vi "Query.vi"(6 "ISOBUS address":T1=-1 caption="ISOBUS address (-1)", 8 "error in":errorcluster, 9 "byte count":u32=4096 caption="byte count (4096)", 10 "Command":string, 11 "Mercury Reference In":T2) -> (0 "error out":errorcluster, 1 "Valid?":bool, 2 "Data":string, 3 "Mercury Reference Out":T2)   [LabVIEW 2019, in "Mercury iXX.lvlib"]
uses:
  Mercury iXX.lvlib
  Public/Controls/Mercury Reference.ctl
  Public/Controls/Comms Transport Layer.ctl
  Controls/Query Dynamic Reference.ctl
  Public/Controls/ISOBus Address.ctl
  <vilib>/Utility/error.llb/whitespace.ctl
  <vilib>/regexp/Match Regular Expression.xnode
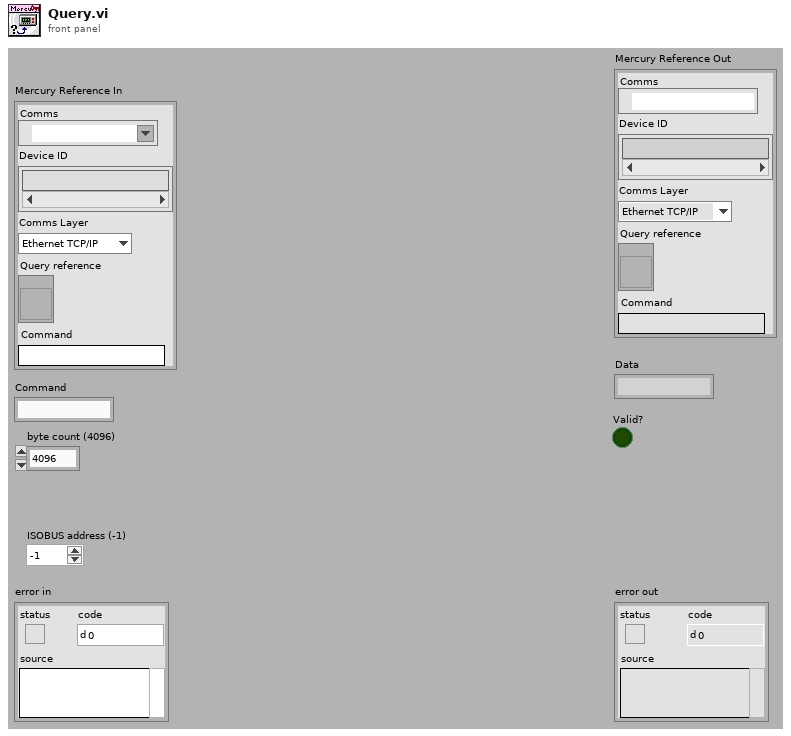
[diagram p1: front panel]
types:
  T1 = typedef "Mercury iXX.lvlib/ISOBus Address.ctl" = i32
  T2 = typedef "Mercury iXX.lvlib/Mercury Reference.ctl" = cluster{"Comms":refnum<visa-resource-name>, "Device ID":string[], "Comms Layer":T3, "Command":string, "Query reference":T4}
  T3 = typedef "Mercury iXX.lvlib/Comms Transport Layer.ctl" = enum16{"Ethernet TCP/IP", "USB", "ISOBus - RS-232", "GPIB"}
  T4 = typedef "Mercury iXX.lvlib/Query Dynamic Reference.ctl" = refnum<vi>
  T5 = typedef "whitespace.ctl" = u16
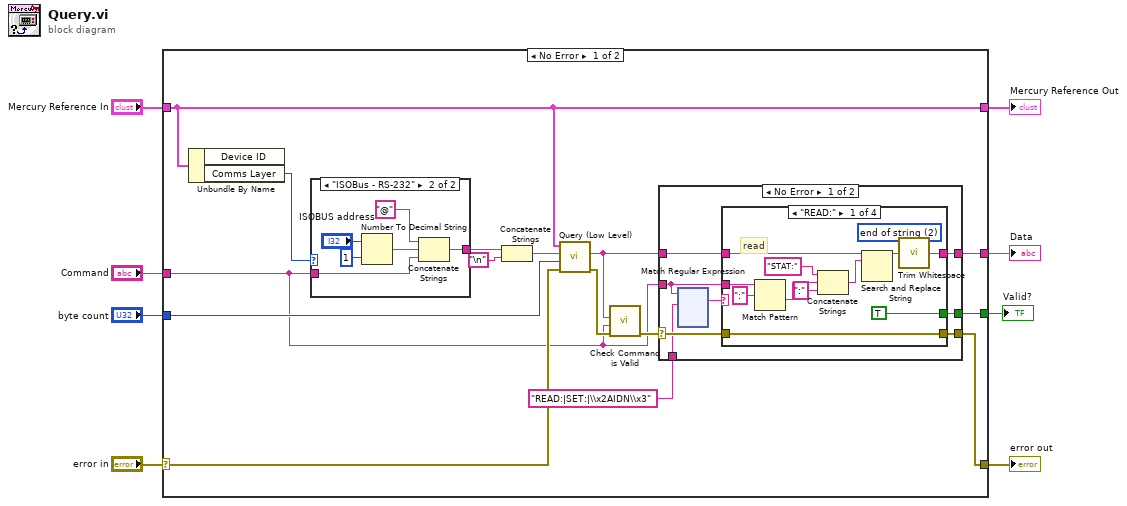
[diagram p0: block diagram]
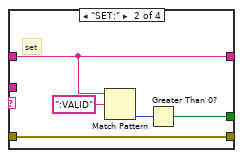
[diagram p2: hidden frame]
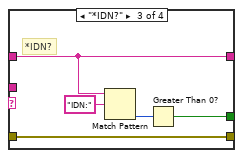
[diagram p3: hidden frame]
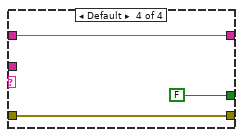
[diagram p4: hidden frame]
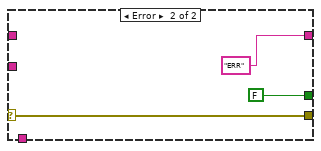
[diagram p5: hidden frame]
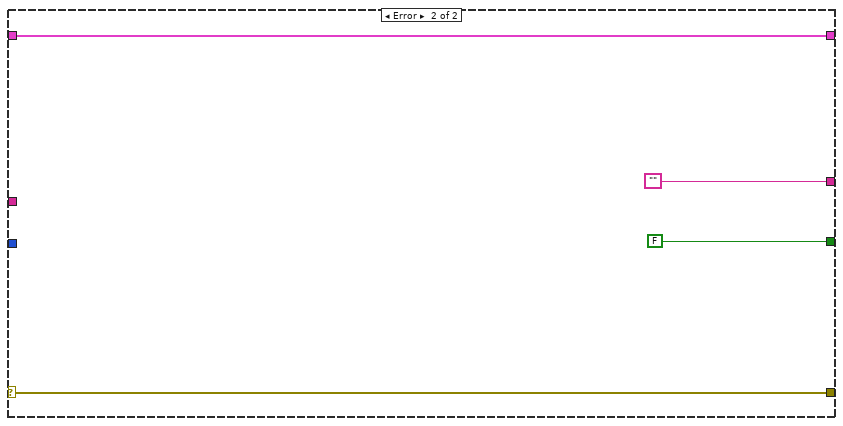
[diagram p7: hidden frame]
diagram:
  n1 = case shown="No Error" "error in" {
    selector: "error in" -> [w20 w184]
    tunnel: [w15 w184] -> w7
    tunnel: "Mercury Reference In" -> [w10 w183]
    tunnel: [w10 w183] -> w5
    tunnel: "Command" -> [w9 _]
    tunnel: [w19 ""] -> w3
    tunnel: "byte count" -> [w14 _]
    tunnel: [w13 FALSE] -> w1
    frame No Error {
      n2 = Unbundle By Name(w10) -> ("Comms Layer"=w11:T3)  [unwired: 1 out]
      n3 = case shown="\"ISOBus - RS-232\"" w11 {
        tunnel: w9 -> [w174 w176]
        tunnel: [w174 w175] -> w22
        frame "Ethernet TCP/IP", Default {
        }
        frame "ISOBus - RS-232" {
          n4 = Number To Decimal String(number="ISOBUS address", width (-)=i16 1) -> (decimal integer string=w178:string)
          n5 = Concatenate Strings("@" ("string"), w178, w176) -> (w175:string)
        }
      }
      n6 = Concatenate Strings(w22, "\n") -> (w21:string)
      n7 = call "Query (Low Level).vi"("error in"=w20, "byte count"=w14, "Command"=w21, "Mercury Reference In"=w10) -> ("error out"=w17:errorcluster, "Response"=w18:string)  [unwired: 1 in, 5 out]
      n8 = call "Check Command is Valid.vi"("error in"=w17, "Cmd Sent"=w9, "Cmd Response"=w18) -> ("error out"=w16:errorcluster)  [unwired: 8 out]
      n9 = case shown="No Error" w16 {
        selector: w16 -> [w30 w172]
        tunnel: w9 -> [w26 _]
        tunnel: [w31 "ERR" ("read buffer")] -> w19
        tunnel: w18 -> [w27 _]
        tunnel: [w29 w172] -> w15
        tunnel: [w28 FALSE] -> w13
        tunnel: "READ:|SET:|\\x2AIDN\\x3" ("regular expression") -> [w25 _]
        frame No Error {
          n10 = xnode "Match Regular Expression"("input string"=w26, "regular expression"=w25) -> ("whole match"=w24:string)  [unwired: 2 in, 6 out]
          n11 = case shown="\"READ:\"" w24 {
            tunnel: [w147 w158 w163 w168] -> w31
            tunnel: w30 -> [w154 w161 w166 w170]
            tunnel: [w154 w161 w166 w170] -> w29
            tunnel: [TRUE w160 w165 FALSE] -> w28
            tunnel: w27 -> [w151 w158 w163 w168]
            tunnel: w26 -> [w152 _ _ _]
            frame "READ:" {
              w146 = T5 2 items=["both", "start of string", "end of string"] ("location (both)")
              # "read"
              n12 = Match Pattern(string=w152, regular expression=":") -> (after substring=w156:string)  [unwired: 4 out]
              n13 = Concatenate Strings("STAT:" ("string"), w156, ":" ("string")) -> (w149:string)
              n14 = Search and Replace String(input string=w151, search string=w149) -> (result string=w150:string)  [unwired: 1 in, 8 out]
              n15 = call <vilib>:"Trim Whitespace.vi"("string"=w150, "location (both)"=w146) -> ("trimmed string"=w147:string)
            }
            frame "SET:" {
              # "set"
              n16 = Match Pattern(string=w158, regular expression=":VALID") -> (offset past match=w159:i32)  [unwired: 4 out]
              n17 = Greater Than 0?(x=w159) -> (x > 0?=w160:bool)
            }
            frame "*IDN?" {
              # "*IDN?"
              n18 = Match Pattern(string=w163, regular expression="IDN:") -> (offset past match=w164:i32)  [unwired: 4 out]
              n19 = Greater Than 0?(x=w164) -> (x > 0?=w165:bool)
            }
            frame Default {
            }
          }
        }
        frame Error {
        }
      }
    }
    frame Error {
    }
  }
  "Mercury Reference Out" <- w5
  "error out" <- w7
  "Data" <- w3
  "Valid?" <- w1
